vi "test_Set-Get Protocol UDP.vi"(8 "error in (no error)":errorcluster, 11 "TestCase in":refnum<class "Instrument Addon Scripting API Custom Device Unit Tests.lvclass">) -> (0 "error out":errorcluster, 3 "TestCase out":refnum<class "Instrument Addon Scripting API Custom Device Unit Tests.lvclass">)   [LabVIEW 2018, in "Instrument Addon Scripting API Custom Device Unit Tests.lvclass"]
uses:
  Instrument Addon Scripting API Custom Device Unit Tests.lvclass
  Addon/Support Libraries/Protocols.lvlibp/UDP/UDP.lvclass
  C:/Users/nitest/Git/NI VS Instrument Addon Fork/Source/Addon/Support Libraries/Protocols.lvlibp/Protocol Parent/Protocol Parent.lvclass
  Addon/Support Libraries/Protocols.lvlibp/TCP/TCP.lvclass
  Addon/Support Libraries/Protocols.lvlibp/UDP/Data Access/Write Local IP Address.vi
  Addon/Support Libraries/Protocols.lvlibp/UDP/Data Access/Write Local Port.vi
  Addon/Support Libraries/Protocols.lvlibp/UDP/Data Access/Write Target IP Address.vi
  Addon/Support Libraries/Protocols.lvlibp/UDP/Data Access/Write Target Port.vi
  Instrument Addon Scripting API Test Assets/Instrument Addon Scripting API Test Assets.lvclass
  <vilib>/addons/_JKI Toolkits/VI Tester/TestCase.llb/TestCase.lvclass
  APIs/Scripting API/Instrument Addon Scripting API.lvlib
  C:/Program Files (x86)/National Instruments/LabVIEW 2018/vi.lib/addons/_JKI Toolkits/VI Tester/TestCase.llb/TestCase.lvclass
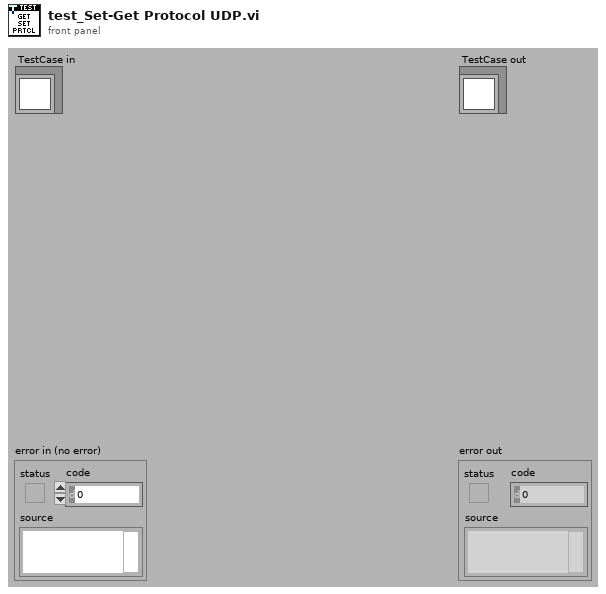
[diagram p1: front panel]
types:
  T1 = typedef "Custom Device API.lvlib/Custom Device Item Ref.ctl" = u64
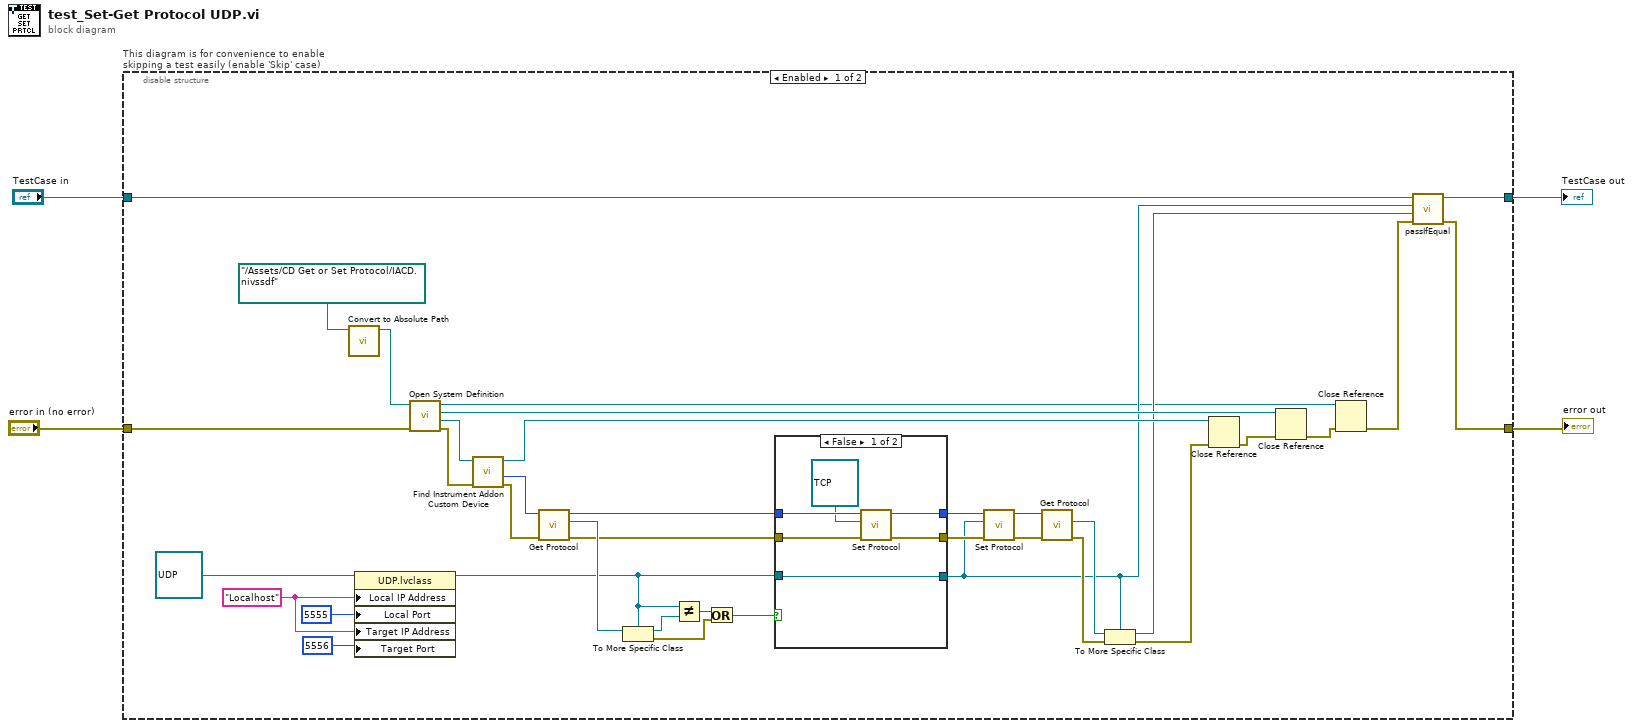
[diagram p0: block diagram]
diagram:
  n1 = disable-structure "This diagram is for convenience to enable skipping a test easily (enable 'Skip' case)" shown="Enabled" {
    disable-tunnel: "TestCase in" -> [w28 w54]
    disable-tunnel: [w27 w52] -> w1
    disable-tunnel: [w24 w53] -> w3
    disable-tunnel: "error in (no error)" -> [w41 w51]
    frame Enabled {
      w20 = "Localhost" ("VISA Resource")
      n2 = call "Convert to Absolute Path.vi"("System Definition File"=path "../Assets/CD Get or Set Protocol/IACD.nivssdf" ("SDF file")) -> ("Absolute Path"=w39:path)  [unwired: 10 in]
      n3 = property class="UDP.lvclass"(reference=refnum<class "UDP.lvclass"> refnum ("Protocols.lvlibp:UDP.lvclass"), "Local IP Address"=w20, "Local Port"=u16 5555, "Target IP Address"=w20, "Target Port"=u16 5556 ("Local Port")) -> (reference out=w8:refnum<class "UDP.lvclass">)  [unwired: 1 in, 1 out]
      n4 = call "Open System Definition.vi"("error in (no error)"=w41, "System Definition File"=w39) -> ("error out"=w36:errorcluster, "Target Refnum"=w35:refnum<k24>, "Root Refnum"=w38:refnum<k24>, "System Definition Refnum"=w6:refnum<k24>)  [unwired: 6 in]
      n5 = call "Find Instrument Addon Custom Device.vi"("error in"=w36, "target in"=w35) -> ("error out"=w19:errorcluster, "NodeID"=w18:u64, "target out"=w34:refnum<k24>)  [unwired: 7 in]
      n6 = call "Get Protocol.vi"("Error In"=w19, "Instrument Addon Refnum In"=w18) -> ("Error Out"=w11:errorcluster, "Protocol"=w14:refnum<class "Protocol Parent.lvclass">, "Instrument Addon Refnum Out"=w12:T1)  [unwired: 7 in]
      n7 = To More Specific Class(target class=w8, reference=w14) -> (specific class reference=w17:refnum<class "UDP.lvclass">, error out=w15:errorcluster)  [unwired: 1 in]
      n8 = Not Equal?(x=w8, y=w17) -> (x != y?=w16:bool)
      n9 = Or(x=w16, y=w15) -> (x .or. y?=w13:bool)
      n10 = case shown="False" w13 {
        tunnel: w12 -> [w45 w50]
        tunnel: w11 -> [w47 w49]
        tunnel: [w46 w49] -> w10
        tunnel: [w43 w50] -> w9
        tunnel: w8 -> [w42 w48]
        tunnel: [w42 w48] -> w7
        frame False {
          n11 = call "Set Protocol.vi"("Error In"=w47, "Protocol in"=refnum<class "TCP.lvclass"> refnum ("Protocols.lvlibp:TCP.lvclass"), "Instrument Addon Refnum In"=w45) -> ("Error Out"=w46:errorcluster, "Instrument Addon Refnum Out"=w43:T1)  [unwired: 7 in]
        }
        frame True {
        }
      }
      n12 = call "Set Protocol.vi"("Error In"=w10, "Protocol in"=w7, "Instrument Addon Refnum In"=w9) -> ("Error Out"=w32:errorcluster, "Instrument Addon Refnum Out"=w33:T1)  [unwired: 7 in]
      n13 = call "Get Protocol.vi"("Error In"=w32, "Instrument Addon Refnum In"=w33) -> ("Error Out"=w30:errorcluster, "Protocol"=w31:refnum<class "Protocol Parent.lvclass">)  [unwired: 7 in, 1 out]
      n14 = To More Specific Class(target class=w7, reference=w31, error in=w30) -> (specific class reference=w26:refnum<class "UDP.lvclass">, error out=w29:errorcluster)
      n15 = Close Reference(reference=w34, error in (no error)=w29) -> (error out=w37:errorcluster)
      n16 = Close Reference(reference=w38, error in (no error)=w37) -> (error out=w5:errorcluster)
      n17 = Close Reference(reference=w6, error in (no error)=w5) -> (error out=w25:errorcluster)
      n18 = call-dynamic "passIfEqual.vi"("error in (no error)"=w25, "y"=w26, "x"=w7, "TestCase in"=w28) -> ("error out"=w24:errorcluster, "TestCase out"=w27:refnum<class "Instrument Addon Scripting API Custom Device Unit Tests.lvclass">)  [unwired: 6 in]
    }
    frame Disabled {
      # "skip test result while test is under development"
      n19 = call <vilib>:"skip.vi"("error in (no error)"=w51, "TestCase in"=w54) -> ("error out"=w53:errorcluster, "TestCase out"=w52:refnum<class "Instrument Addon Scripting API Custom Device Unit Tests.lvclass">)  [unwired: 8 in]
    }
  }
  "error out" <- w3
  "TestCase out" <- w1
